vi "Load Ramp Time.vi"(4 "Ramp Type String":string, 5 "error in (no error)":errorcluster, 6 "refnum":T2, 7 "Input Cluster":T1, 8 "section":string) -> (0 "error out":errorcluster, 2 "output cluster":T1, 3 "refnum out":T2)   [LabVIEW 2013]
uses:
  MixedMode/Ramp Control.ctl
  <vilib>/Utility/config.llb/Config Data RefNum.ctl
  <vilib>/Utility/config.llb/Read Key (Double).vi
  <vilib>/Utility/config.llb/NI_LVConfig.lvlib
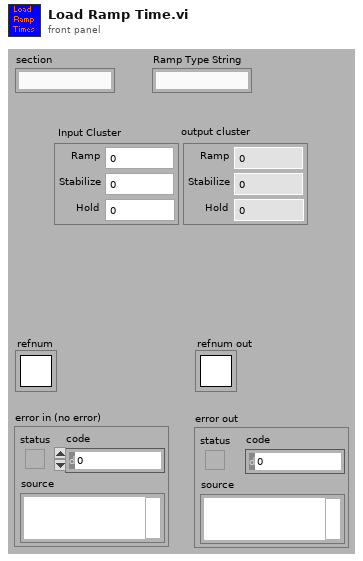
[diagram p1: front panel]
types:
  T1 = typedef "Ramp Control.ctl" = cluster{"Ramp":dbl, "Stabilize":dbl, "Hold":dbl}
  T2 = typedef "NI_LVConfig.lvlib/Config Data RefNum.ctl" = refnum<k1>
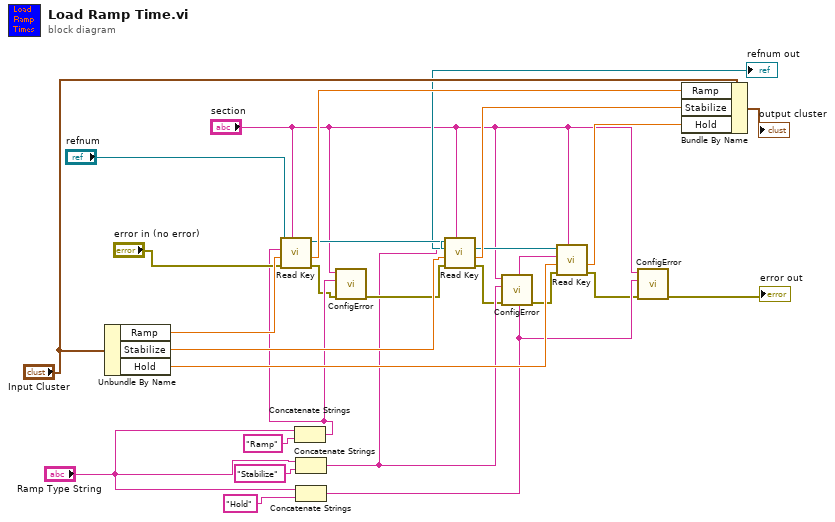
[diagram p0: block diagram]
diagram:
  n1 = Unbundle By Name("Input Cluster") -> ("Ramp"=w21:dbl, "Stabilize"=w22:dbl, "Hold"=w23:dbl)
  n2 = Concatenate Strings("Ramp Type String", "Ramp" ("string")) -> (w10:string)
  n3 = call-poly <vilib>:"Read Key.vi"("section"="section", "error in (no error)"="error in (no error)", "default value"=w21, "key"=w10, "refnum"="refnum") -> ("error out"=w9:errorcluster, "value"=w25:dbl, "refnum out"=w18:T2)  [unwired: 4 out]
  n4 = Concatenate Strings("Ramp Type String", "Stabilize" ("string")) -> (w7:string)
  n5 = Concatenate Strings("Ramp Type String", "Hold" ("string")) -> (w3:string)
  n6 = call "ConfigError.vi"("error in (no error)"=w9, "Key"=w10, "Section"="section") -> ("error out"=w8:errorcluster)  [unwired: 8 out]
  n7 = call-poly <vilib>:"Read Key.vi"("section"="section", "error in (no error)"=w8, "default value"=w22, "key"=w7, "refnum"=w18) -> ("error out"=w6:errorcluster, "value"=w26:dbl, "refnum out"=w20:T2)  [unwired: 4 out]
  n8 = call "ConfigError.vi"("error in (no error)"=w6, "Key"=w7, "Section"="section") -> ("error out"=w5:errorcluster)  [unwired: 8 out]
  n9 = call-poly <vilib>:"Read Key.vi"("section"="section", "error in (no error)"=w5, "default value"=w23, "key"=w3, "refnum"=w20) -> ("error out"=w2:errorcluster, "value"=w27:dbl, "refnum out"=→"refnum out":T2)  [unwired: 4 out]
  n10 = call "ConfigError.vi"("error in (no error)"=w2, "Key"=w3, "Section"="section") -> ("error out"=→"error out":errorcluster)  [unwired: 8 out]
  n11 = Bundle By Name(cluster="Input Cluster", "Ramp"=w25, "Stabilize"=w26, "Hold"=w27) -> (→"output cluster":T1)
